vi "Get ESP.vi"(8 "error in (no error)":errorcluster, 11 "Sabritas Actor in":refnum<class "Sabritas Actor.lvclass">) -> (0 "error out":errorcluster, 2 "ESP":bool, 3 "Sabritas Actor out":refnum<class "Sabritas Actor.lvclass">)   [LabVIEW 2020, in "Sabritas Actor.lvlib" / "Sabritas Actor.lvclass"]
uses:
  Sabritas Actor.lvclass
  Sabritas Actor.lvclass/Sabritas Actor.ctl
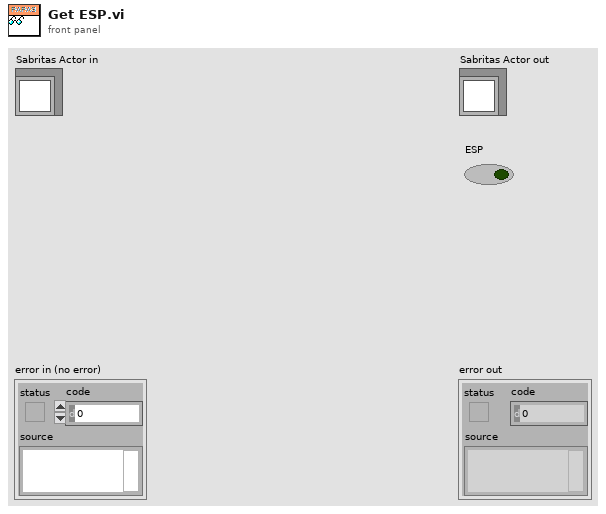
[diagram p1: front panel]
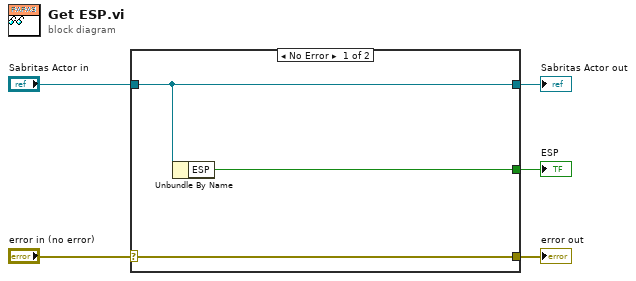
[diagram p0: block diagram]
diagram:
  n1 = case shown="No Error" "error in (no error)" {
    selector: "error in (no error)" -> [w8 w9]
    tunnel: [w8 w9] -> w4
    tunnel: [w7 w10] -> w2
    tunnel: "Sabritas Actor in" -> [w7 w10]
    tunnel: [w6 _] -> w1
    frame No Error {
      n2 = Unbundle By Name(w7) -> ("ESP"=w6:bool)
    }
    frame Error {
    }
  }
  "error out" <- w4
  "Sabritas Actor out" <- w2
  "ESP" <- w1
